vi "F510-D.vi"(8 "error in (no error)":errorcluster, 10 "Deadzone Scale Cluster":cluster{"Scale":dbl, "Deadzone":dbl}={"Scale"=1.0, "Deadzone"=0.1}, 11 "refnum name":string) -> (0 "error out":errorcluster, 1 "D-Pad Buttons":T1, 2 "Right Stick":cluster{"X":dbl, "Y":dbl}, 3 "Left Stick":cluster{"X":dbl, "Y":dbl}, 4 "Buttons":T2)   [LabVIEW 2014]
uses:
  <vilib>/Rock Robotics/WPI/Joystick/WPI_JoystickGetSetRefNum.vi
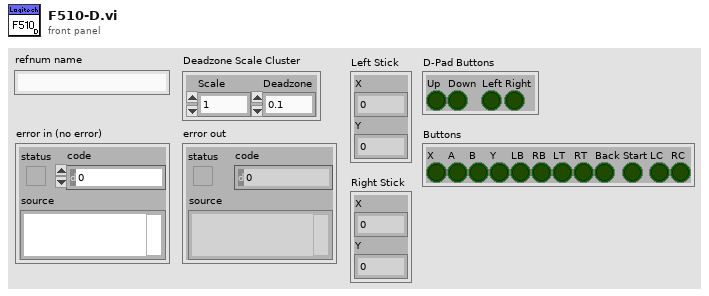
[diagram p1: front panel]
types:
  T1 = cluster{"Up":bool, "Down":bool, "Left":bool, "Right":bool}
  T2 = cluster{"X":bool, "A":bool, "B":bool, "Y":bool, "LB":bool, "RB":bool, "LT":bool, "RT":bool, "Back":bool, "Start":bool, "LC":bool, "RC":bool}
  T3 = typedef "WPI_JoystickDevRef.ctl" = cluster{"Device":T4}
  T4 = typedef "WPI_JoystickDeviceEnum.ctl" = enum16{"USB 0", "USB 1", "USB 2", "USB 3", "USB 4", "USB 5"}
  T5 = cluster{"Up":bool, "Down":bool, "Left":bool, "Right":bool}[]
  T6 = cluster{"Buttons[0]":bool, "Buttons[1]":bool, "Buttons[2]":bool, "Buttons[3]":bool, "Buttons[4]":bool, "Buttons[5]":bool, "Buttons[6]":bool, "Buttons[7]":bool, "Buttons[8]":bool, "Buttons[9]":bool, "Buttons[10]":bool, "Buttons[11]":bool}
  T7 = cluster{"[0]":dbl, "[1]":dbl, "[2]":dbl, "[3]":dbl}
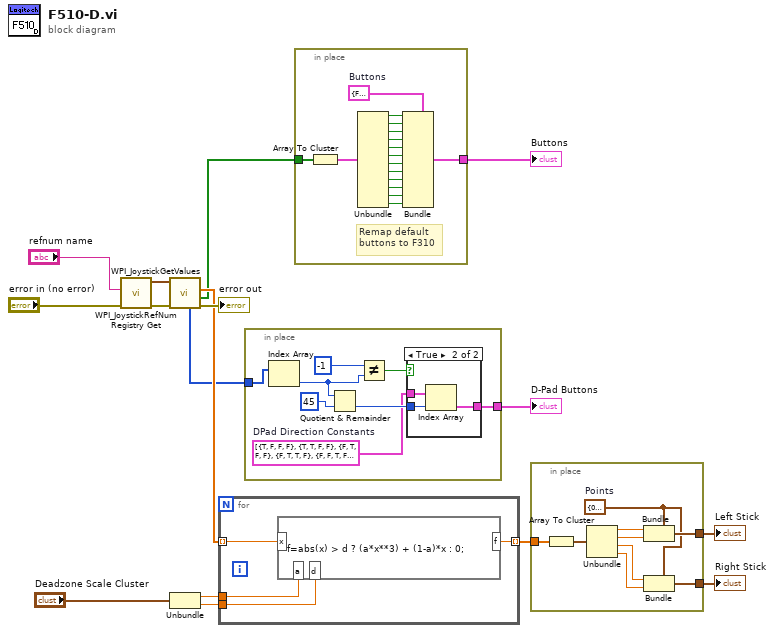
[diagram p0: block diagram]
diagram:
  n1 = call <vilib>:"WPI_JoystickRefNum Registry Get.vi"("error in (no error)"="error in (no error)", "refnum name"="refnum name") -> ("error out"=w13:errorcluster, "JoystickDevRef"=w14:T3)  [unwired: 8 in]
  n2 = call <vilib>:"WPI_JoystickGetValues.vi"("error in (no error)"=w13, "JoystickDevRef"=w14) -> ("error out"=→"error out":errorcluster, "Buttons"=w3:bool[], "Axes"=w11:dbl[], "POVs"=w2:i16[])  [unwired: 5 in, 1 out]
  n3 = Unbundle("Deadzone Scale Cluster") -> ("Scale"=w9:dbl, "Deadzone"=w8:dbl)
  n4 = for {
    tunnel: w11 -> [w20] mode=indexing
    tunnel: w9 -> [w19]
    tunnel: w8 -> [w18]
    tunnel: [w17] -> w7 mode=indexing
    n5 = formula code="f=abs(x) > d ? (a*x**3) + (1-a)*x : 0;"("x"=w20, "d"=w18, "a"=w19) -> ("f"=w17:dbl)
  }
  n6 = in-place {
    in-place-border: w2 -> [w28]
    in-place-border: [w23] -> w1
    w24 = T5 [{"Up"=TRUE, "Down"=FALSE, "Left"=FALSE, "Right"=FALSE}, {"Up"=TRUE, "Down"=TRUE, "Left"=FALSE, "Right"=FALSE}, {"Up"=FALSE, "Down"=TRUE, "Left"=FALSE, "Right"=FALSE}, {"Up"=FALSE, "Down"=TRUE, "Left"=TRUE, "Right"=FALSE}, {"Up"=FALSE, "Down"=FALSE, "Left"=TRUE, "Right"=FALSE}, {"Up"=FALSE, "Down"=FALSE, "Left"=TRUE, "Right"=TRUE}, {"Up"=FALSE, "Down"=FALSE, "Left"=FALSE, "Right"=TRUE}, {"Up"=TRUE, "Down"=FALSE, "Left"=FALSE, "Right"=TRUE}]  # DPad Direction Constants
    n7 = Index Array(array=w28) -> (element=w22:i16)  [unwired: 1 in]
    n8 = Quotient & Remainder(x=w22, y=u16 45) -> (floor(x/y)=w26:u16)  [unwired: 1 out]
    n9 = Not Equal?(x=i16 -1, y=w22) -> (x != y?=w25:bool)
    n10 = case shown="True" w25 {
      tunnel: w26 -> [_ w31]
      tunnel: w24 -> [_ w30]
      tunnel: [_ w29] -> w23
      frame False {
      }
      frame True {
        n11 = Index Array(array=w30, index=w31) -> (element=w29:T1)
      }
    }
  }
  "D-Pad Buttons" <- w1
  n12 = in-place {
    in-place-border: w3 -> [w32]
    in-place-border: [w34] -> w4
    w47 = T2 {"X"=FALSE, "A"=FALSE, "B"=FALSE, "Y"=FALSE, "LB"=FALSE, "RB"=FALSE, "LT"=FALSE, "RT"=FALSE, "Back"=FALSE, "Start"=FALSE, "LC"=FALSE, "RC"=FALSE}  # Buttons
    # "Remap default\nbuttons to F310"
    n13 = Array To Cluster(array=w32) -> (cluster=w33:T6)
    n14 = Unbundle(w33) -> ("Buttons[0]"=w46:bool, "Buttons[1]"=w45:bool, "Buttons[2]"=w44:bool, "Buttons[3]"=w43:bool, "Buttons[4]"=w42:bool, "Buttons[5]"=w41:bool, "Buttons[6]"=w40:bool, "Buttons[7]"=w39:bool, "Buttons[8]"=w38:bool, "Buttons[9]"=w37:bool, "Buttons[10]"=w36:bool, "Buttons[11]"=w35:bool)
    n15 = Bundle(cluster=w47, "X"=w46, "A"=w45, "B"=w44, "Y"=w43, "LB"=w42, "RB"=w41, "LT"=w40, "RT"=w39, "Back"=w38, "Start"=w37, "LC"=w36, "RC"=w35) -> (w34:T2)
  }
  "Buttons" <- w4
  n16 = in-place {
    in-place-border: w7 -> [w51]
    in-place-border: [w50] -> w5
    in-place-border: [w49] -> w6
    w48 = cluster{"X":dbl, "Y":dbl} {"X"=0.0, "Y"=0.0}  # Points
    n17 = Array To Cluster(array=w51) -> (cluster=w56:T7)
    n18 = Unbundle(w56) -> ("[0]"=w52:dbl, "[1]"=w53:dbl, "[2]"=w54:dbl, "[3]"=w55:dbl)
    n19 = Bundle(cluster=w48, "X"=w52, "Y"=w53) -> (w49:cluster{"X":dbl, "Y":dbl})
    n20 = Bundle(cluster=w48, "X"=w54, "Y"=w55) -> (w50:cluster{"X":dbl, "Y":dbl})
  }
  "Left Stick" <- w6
  "Right Stick" <- w5
